vi "Final Webcam.vi"(1 "stop":bool) -> (0 "Live Stream":T1(plugin-control))   [LabVIEW 2017]
uses:
  <vilib>/vision/Avi.llb/IMAQ AVI2 Refnum.ctl
  <vilib>/userdefined/High Color/IMAQdx.ctl
  <vilib>/vision/driver/NI_Vision_Acquisition_Software.lvlib
  <resource>/objmgr/imaqdx.rc
panel:
  out "Clock 2":cluster{dbl, dbl, dbl}(knob)={0.0, 1.701440214160589, 1.7350906402478021} scale=0.012..12.0
  out "Clock":cluster{dbl, dbl, dbl}(knob)={0.0, 1.701440214160589, 1.7350906402478021} scale=0.012..12.0
  out "# of Pics":dbl
  in  "Snap Picture":bool
  out "path":path
  in  "Record":bool
  out "stop 2":bool
  out "AVI Refnum":T2
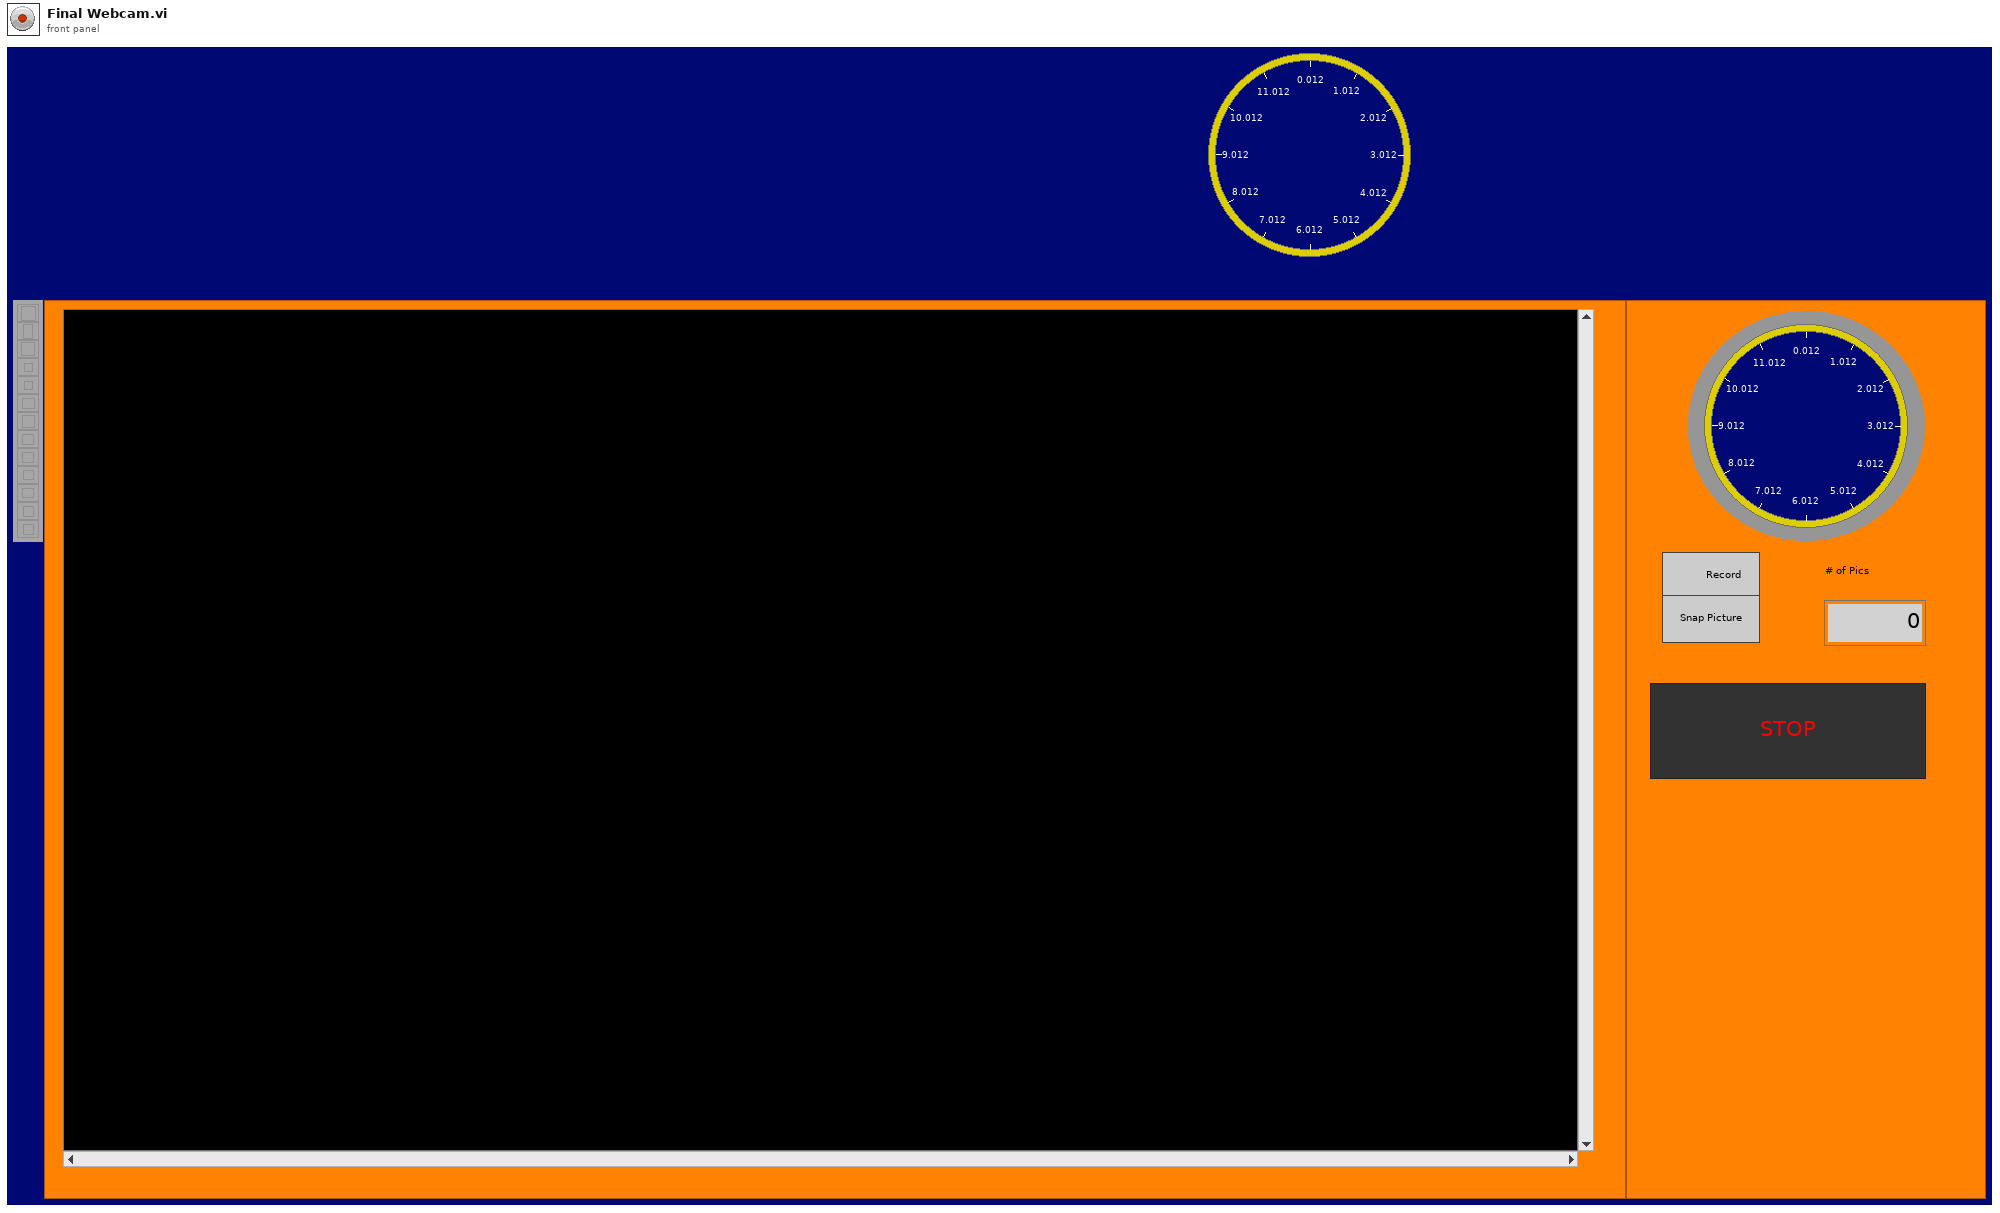
[diagram p1: front panel]
types:
  T1 = typedef "IMAQ Image.ctl" = refnum<image>
  T2 = typedef "IMAQ AVI2 Refnum.ctl" = refnum<k20>
  T3 = typedef "LVDateTimeRec.ctl" = cluster{"fractional second":dbl, "second":i32, "minute":i32, "hour":i32, "day of month":i32, "month":i32, "year":i32, "day of week":i32, "day of year":i32, "DST":i32}
  T4 = typedef "IMAQdx.ctl" = refnum<k21>
  T5 = typedef "Image Type" = u32
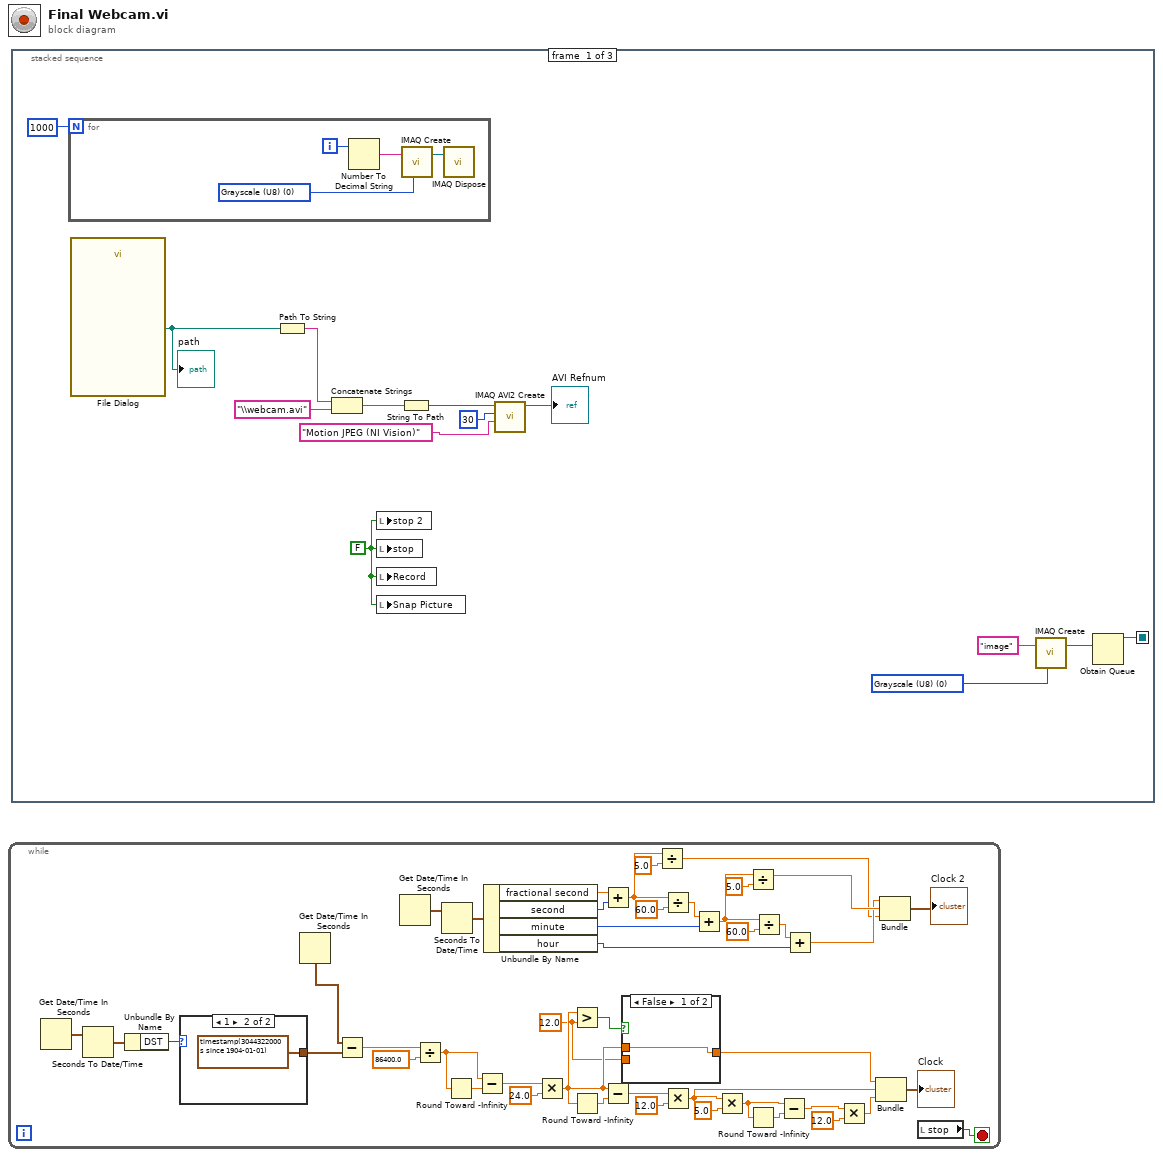
[diagram p0: block diagram]
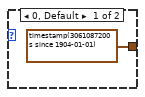
[diagram p2: hidden frame]
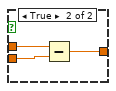
[diagram p3: hidden frame]
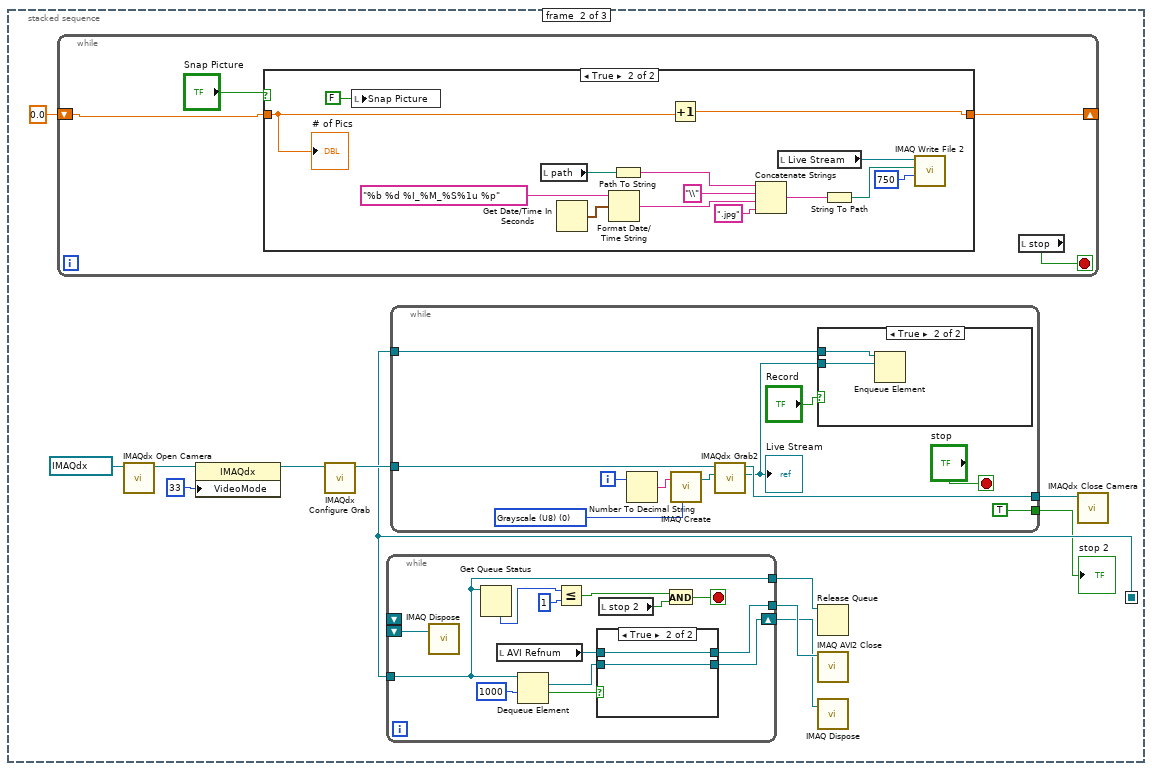
[diagram p4: hidden frame]
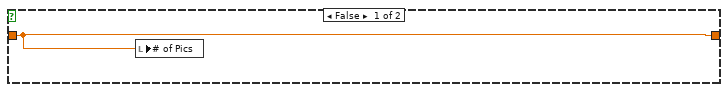
[diagram p5: hidden frame]
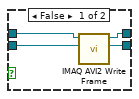
[diagram p6: hidden frame]
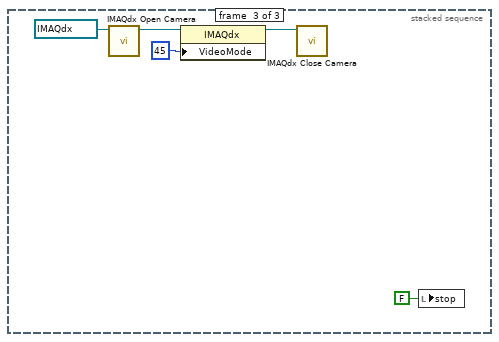
[diagram p8: hidden frame]
diagram:
  n1 = while {
    stop <- w19 stop-if-true
    w22 = 12.0 ("y")
    n2 = Get Date/Time In Seconds() -> (seconds since 1Jan1904=w44:timestamp)
    n3 = Seconds To Date/Time(time stamp (now)=w44) -> (date time rec=w43:T3)  [unwired: 1 in]
    n4 = Unbundle By Name(w43) -> ("DST"=w45:i32)
    n5 = case shown="1" w45 {
      tunnel: [timestamp(3061087200 s since 1904-01-01) ("y") timestamp(3044322000 s since 1904-01-01) ("y")] -> w27
      frame 0, Default {
      }
      frame 1 {
      }
    }
    n6 = Get Date/Time In Seconds() -> (seconds since 1Jan1904=w26:timestamp)
    n7 = Subtract(x=w26, y=w27) -> (x-y=w28:dbl)
    n8 = Get Date/Time In Seconds() -> (seconds since 1Jan1904=w15:timestamp)
    n9 = Divide(x=w28, y=86400.0) -> (x/y=w29:dbl)
    n10 = Seconds To Date/Time(time stamp (now)=w15) -> (date time rec=w16:T3)  [unwired: 1 in]
    n11 = Round Toward -Infinity(1:w29) -> (0:w30:dbl)
    n12 = Subtract(x=w29, y=w30) -> (x-y=w31:dbl)
    n13 = Unbundle By Name(w16) -> ("fractional second"=w17:dbl, "second"=w18:i32, "minute"=w11:i32, "hour"=w4:i32)
    n14 = Multiply(x=w31, y=24.0) -> (x*y=w35:dbl)
    n15 = Greater?(x=w35, y=w22) -> (0:w32:bool)
    n16 = Round Toward -Infinity(1:w35) -> (0:w34:dbl)
    n17 = Add(x=w17, y=w18) -> (x+y=w14:dbl)
    n18 = Subtract(x=w35, y=w34) -> (x-y=w36:dbl)
    n19 = case shown="False" w32 {
      tunnel: [w48 w51] -> w33
      tunnel: w35 -> [w48 w50]
      tunnel: w22 -> [_ w49]
      frame False {
      }
      frame True {
        n20 = Subtract(x=w50, y=w49) -> (x-y=w51:dbl)
      }
    }
    n21 = Divide(x=w14, y=5.0) -> (x/y=w1:dbl)
    n22 = Divide(x=w14, y=60.0) -> (x/y=w12:dbl)
    n23 = Multiply(x=w36, y=12.0) -> (x*y=w37:dbl)
    n24 = Add(x=w12, y=w11) -> (x+y=w7:dbl)
    n25 = Multiply(x=w37, y=5.0) -> (x*y=w39:dbl)
    n26 = Divide(x=w7, y=5.0) -> (x/y=w8:dbl)
    n27 = Round Toward -Infinity(1:w39) -> (0:w38:dbl)
    n28 = Divide(x=w7, y=60.0) -> (x/y=w5:dbl)
    n29 = Subtract(x=w39, y=w38) -> (x-y=w40:dbl)
    n30 = Add(x=w5, y=w4) -> (x+y=w2:dbl)
    n31 = Multiply(x=w40, y=12.0) -> (x*y=w41:dbl)
    n32 = Bundle(w33, w37, w41) -> (→"Clock":cluster{dbl, dbl, dbl})  [unwired: 1 in]
    n33 = Bundle(w2, w8, w1) -> (→"Clock 2":cluster{dbl, dbl, dbl})  [unwired: 1 in]
    n34 = local read "stop"() -> (w19:bool)
  }
  n35 = stacked-sequence {
    seq-local: [w58 _ _] -> [_ w77 _]
    frame #0 {
      w52 = FALSE
      w60 = T5 0 items=["Grayscale (U8)", "Grayscale (I16)", "Grayscale (SGL)", "Complex (CSG)", "RGB (U32)", "HSL (U32)", "RGB (U64)", "Grayscale (U16)"] ("Image Type")
      n36 = for {
        N: 1000 -> [_]
        i -> [w69]
        w66 = T5 0 items=["Grayscale (U8)", "Grayscale (I16)", "Grayscale (SGL)", "Complex (CSG)", "RGB (U32)", "HSL (U32)", "RGB (U64)", "Grayscale (U16)"] ("Image Type")
        n37 = Number To Decimal String(number=w69) -> (decimal integer string=w68:string)  [unwired: 1 in]
        n38 = call "IMAQ Create"("Image Name"=w68, "Image Type"=w66) -> ("New Image"=w67:T1)  [unwired: 3 in, 1 out]
        n39 = call "IMAQ Dispose"("Image"=w67) -> ()  [unwired: 5 in, 1 out]
      }
      n40 = call "File Dialog"() -> ("selected path"=w53:path)  [unwired: 12 in, 3 out]
      "path" <- w53
      n41 = Path To String(path=w53) -> (string=w57:string)
      n42 = Concatenate Strings(w57, "\\webcam.avi" ("string")) -> (w55:string)
      n43 = local write "stop 2"(w52) -> ()
      n44 = local write "stop"(w52) -> ()
      n45 = local write "Record"(w52) -> ()
      n46 = local write "Snap Picture"(w52) -> ()
      n47 = String To Path(string=w55) -> (path=w54:path)
      n48 = call "IMAQ AVI2 Create"("Codec"="Motion JPEG (NI Vision)", "Frames Per Second"=u32 30, "AVI Path"=w54) -> ("AVI Refnum"=→"AVI Refnum":T2)  [unwired: 7 in, 1 out]
      n49 = call "IMAQ Create"("Image Name"="image", "Image Type"=w60) -> ("New Image"=w61:T1)  [unwired: 3 in, 1 out]
      n50 = Obtain Queue(element data type=w61) -> (queue out=w58:refnum<queue>)  [unwired: 4 in, 2 out]
    }
    frame #1 {
      n51 = while {
        shift-right: [w82] -> _
        shift-left: 0.0 -> [w83]
        stop <- w84 stop-if-true
        n52 = case shown="True" "Snap Picture" {
          tunnel: w83 -> [w86 w89]
          tunnel: [w86 w88] -> w82
          frame False {
            n53 = local write "# of Pics"(w86) -> ()
          }
          frame True {
            n54 = local write "Snap Picture"(FALSE) -> ()
            n55 = local read "path"() -> (w99:path)
            n56 = Get Date/Time In Seconds() -> (seconds since 1Jan1904=w100:timestamp)
            n57 = Format Date/Time String(time format string (%c)="%b %d %I_%M_%S%1u %p", seconds (now)=w100) -> (date/time string=w91:string)  [unwired: 1 in]
            n58 = Path To String(path=w99) -> (string=w93:string)
            n59 = Increment(x=w89) -> (x+1=w88:dbl)
            n60 = Concatenate Strings(w93, "\\" ("string"), w91, ".jpg" ("string")) -> (w90:string)
            n61 = local read "Live Stream"() -> (w94:T1)
            n62 = String To Path(string=w90) -> (path=w95:path)
            n63 = call-poly "IMAQ Write File 2"("Image Quality"=u32 750, "File Path"=w95, "Image"=w94) -> ()  [unwired: 7 in, 2 out]
            "# of Pics" <- w89
          }
        }
        n64 = local read "stop"() -> (w84:bool)
      }
      n65 = call <vilib>:"IMAQdx Open Camera.vi"("Session In"=T4 "cam10") -> ("Session Out"=w70:T4)  [unwired: 9 in, 1 out]
      n66 = property class="IMAQdx"(reference=w70, "VideoMode"=u32 33) -> (reference out=w71:T4)  [unwired: 1 in, 1 out]
      n67 = call <vilib>:"IMAQdx Configure Grab.vi"("Session In"=w71) -> ("Session Out"=w81:T4)  [unwired: 9 in, 1 out]
      n68 = while {
        tunnel: [w110] -> w75
        tunnel: [w106] -> w76
        tunnel: w77 -> [w106]
        shift-right: [w102] -> w73
        shift-left: _ -> [_]
        shift-left: _ -> [w101]
        stop <- w107 stop-if-true
        n69 = call "IMAQ Dispose"("Image"=w101) -> ()  [unwired: 5 in, 1 out]
        n70 = Get Queue Status(queue=w106) -> (# elements in queue=w111:i32)  [unwired: 2 in, 7 out]
        n71 = local read "AVI Refnum"() -> (w113:T2)
        n72 = Dequeue Element(queue=w106, timeout in ms (-1)=1000) -> (element=w109:T1, timed out?=w103:bool)  [unwired: 1 in, 2 out]
        n73 = Less Or Equal?(x=w111, y=1) -> (x <= y?=w108:bool)
        n74 = case shown="True" w103 {
          tunnel: w113 -> [w117 w119]
          tunnel: [w116 w119] -> w110
          tunnel: w109 -> [w115 w118]
          tunnel: [w114 w118] -> w102
          frame False {
            n75 = call "IMAQ AVI2 Write Frame"("Image"=w115, "AVI Refnum"=w117) -> ("Image Out (duplicate)"=w114:T1, "AVI Refnum (duplicate)"=w116:T2)  [unwired: 7 in, 1 out]
          }
          frame True {
          }
        }
        n76 = local read "stop 2"() -> (w105:bool)
        n77 = And(x=w108, y=w105) -> (x .and. y?=w107:bool)
      }
      n78 = while {
        tunnel: w81 -> [w130]
        tunnel: [w125] -> w78
        tunnel: w77 -> [w123]
        tunnel: [TRUE] -> w74
        i -> [w129]
        stop <- "stop" stop-if-true
        w124 = T5 0 items=["Grayscale (U8)", "Grayscale (I16)", "Grayscale (SGL)", "Complex (CSG)", "RGB (U32)", "HSL (U32)", "RGB (U64)", "Grayscale (U16)"] ("Image Type")
        n79 = Number To Decimal String(number=w129) -> (decimal integer string=w128:string)  [unwired: 1 in]
        n80 = call "IMAQ Create"("Image Name"=w128, "Image Type"=w124) -> ("New Image"=w127:T1)  [unwired: 3 in, 1 out]
        n81 = call <vilib>:"IMAQdx Grab2.vi"("Image In"=w127, "Session In"=w130) -> ("Image Out"=w120:T1, "Session Out"=w125:T4)  [unwired: 6 in, 2 out]
        "Live Stream" <- w120
        n82 = case shown="True" "Record" {
          tunnel: w123 -> [_ w132]
          tunnel: w120 -> [_ w131]
          frame False {
          }
          frame True {
            n83 = Enqueue Element(queue=w132, element=w131) -> ()  [unwired: 2 in, 3 out]
          }
        }
      }
      "stop 2" <- w74
      n84 = Release Queue(queue=w76) -> ()  [unwired: 2 in, 3 out]
      n85 = call "IMAQ AVI2 Close"("AVI Refnum"=w75) -> ()  [unwired: 10 in, 1 out]
      n86 = call "IMAQ Dispose"("Image"=w73) -> ()  [unwired: 5 in, 1 out]
      n87 = call <vilib>:"IMAQdx Close Camera.vi"("Session In"=w78) -> ()  [unwired: 10 in, 1 out]
    }
    frame #2 {
      n88 = call <vilib>:"IMAQdx Open Camera.vi"("Session In"=T4 "cam10") -> ("Session Out"=w136:T4)  [unwired: 9 in, 1 out]
      n89 = property class="IMAQdx"(reference=w136, "VideoMode"=u32 45) -> (reference out=w134:T4)  [unwired: 1 in, 1 out]
      n90 = call <vilib>:"IMAQdx Close Camera.vi"("Session In"=w134) -> ()  [unwired: 10 in, 1 out]
      n91 = local write "stop"(FALSE ("stop")) -> ()
    }
  }
